vi "AMZ_S3_APIHLP_Parse RequestPayentConfiguration.vi"(8 "error in (no error)":errorcluster, 10 "Response body":string) -> (0 "error out":errorcluster, 3 "RequestPaymentConfiguration":T1)   [LabVIEW 2015, in "LV Interface for Amazon S3.lvlib"]
uses:
  LV Interface for Amazon S3.lvlib
  Typedefs/AMZ_S3_API_RequestPaymentConfig.ctl
  Typedefs/AMZ_S3_Payer.ctl
  XML Parser/XML Parser.lvlib
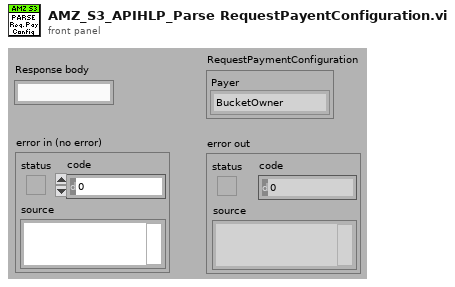
[diagram p1: front panel]
types:
  T1 = typedef "LV Interface for Amazon S3.lvlib/AMZ_S3_API_RequestPaymentConfig.ctl" = cluster{"Payer":T2}
  T2 = typedef "LV Interface for Amazon S3.lvlib/AMZ_S3_Payer.ctl" = enum16{"BucketOwner", "Requester"}
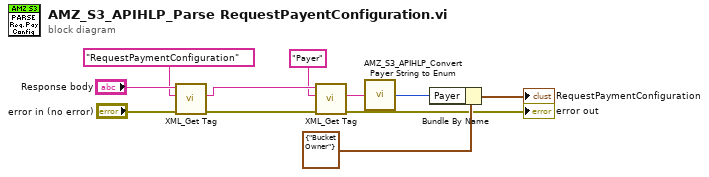
[diagram p0: block diagram]
diagram:
  n1 = call "XML_Get Tag.vi"("error in (no error)"="error in (no error)", "Tag name"="RequestPaymentConfiguration", "XML String in"="Response body") -> ("error out"=w8:errorcluster, "Tag value"=w7:string)  [unwired: 4 in, 3 out]
  n2 = call "XML_Get Tag.vi"("error in (no error)"=w8, "Tag name"="Payer", "XML String in"=w7) -> ("error out"=→"error out":errorcluster, "Tag value"=w5:string)  [unwired: 4 in, 3 out]
  n3 = call "AMZ_S3_APIHLP_Convert Payer String to Enum.vi"("Payer String"=w5) -> ("Payer"=w3:T2)  [unwired: 4 in]
  n4 = Bundle By Name(cluster=T1 {"Payer"=enum."BucketOwner"} ("RequestPaymentConfiguration"), "Payer"=w3) -> (→"RequestPaymentConfiguration":T1)
